vi "[GV]_Vision Lane.vi"() -> ()   [LabVIEW 2016, in "Vision Variables.lvlib"]
uses:
  Vision Variables.lvlib
panel:
  out "Lane":dbl[][](array[numeric])
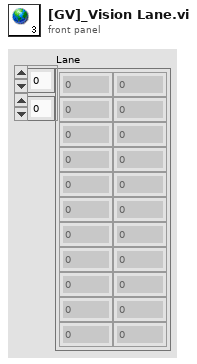
[diagram p1: front panel]
diagram:
